vi "集成干预.vi"(11 "数据标记表":string(combo)="N") -> ()   [LabVIEW 2016, in "斯坦道多参数.lvlib"]
panel:
  out "运行状态":u16(ring) items=["空闲", "水样测试", "标样核查"]
  out "多参数运行日志":string
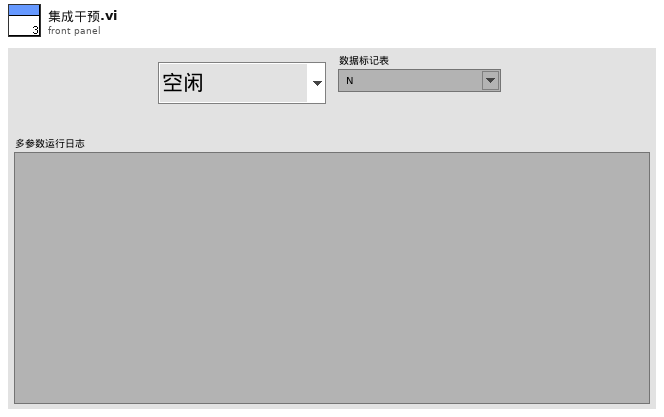
[diagram p1: front panel]
types:
  T1 = typedef "集成多参数单参数字段定义.ctl" = cluster{"时间":timestamp, "测量模式":string, "数据类型":string, "检测值":sgl, "单位":string, "数据标识":string, "标样参考值":sgl, "因子编码":string, "LastTime":timestamp}
  T2 = cluster{"水温":bool, "pH":bool, "DO":bool, "DOper":bool, "电导率":bool, "ORP":bool, "浊度":bool, "叶绿素a":bool, "藻密度":bool, "COD":bool, "DO2":bool, "DOper":bool, "氯化物":bool, "氨氮":bool, "水中油":bool}
  T3 = cluster{"ph":bool, "DO":bool, "Cond":bool, "Turb":bool, "叶绿素a":bool, "藻密度":bool, "ORP":bool, "cod":bool, "DO2":bool, "氯化物":bool, "氨氮":bool, "水中油":bool}
  T4 = cluster{"温度测量值":sgl, "测量值":sgl, "温度偏移修正值":sgl, "信号值":sgl, "数据标识":string}
  T5 = cluster{"温度测量值":sgl, "DO%":sgl, "DOmg/L":sgl, "温度偏移修正值":sgl, "数据标识mg/L":string, "数据标识%":string}
  T6 = cluster{"CH":u16, "监测值":dbl, "信号值":sgl, "数据标识":string}
  T7 = cluster{"水样数据时间":timestamp, "水温":dbl, "pH":dbl, "DO":dbl, "DOper":dbl, "电导率":dbl, "ORP":dbl, "浊度":dbl, "叶绿素a":dbl, "藻密度":dbl, "COD":dbl, "DO2":dbl, "DO2per":dbl, "氯化物":dbl, "氨氮":dbl, "水中油":dbl}
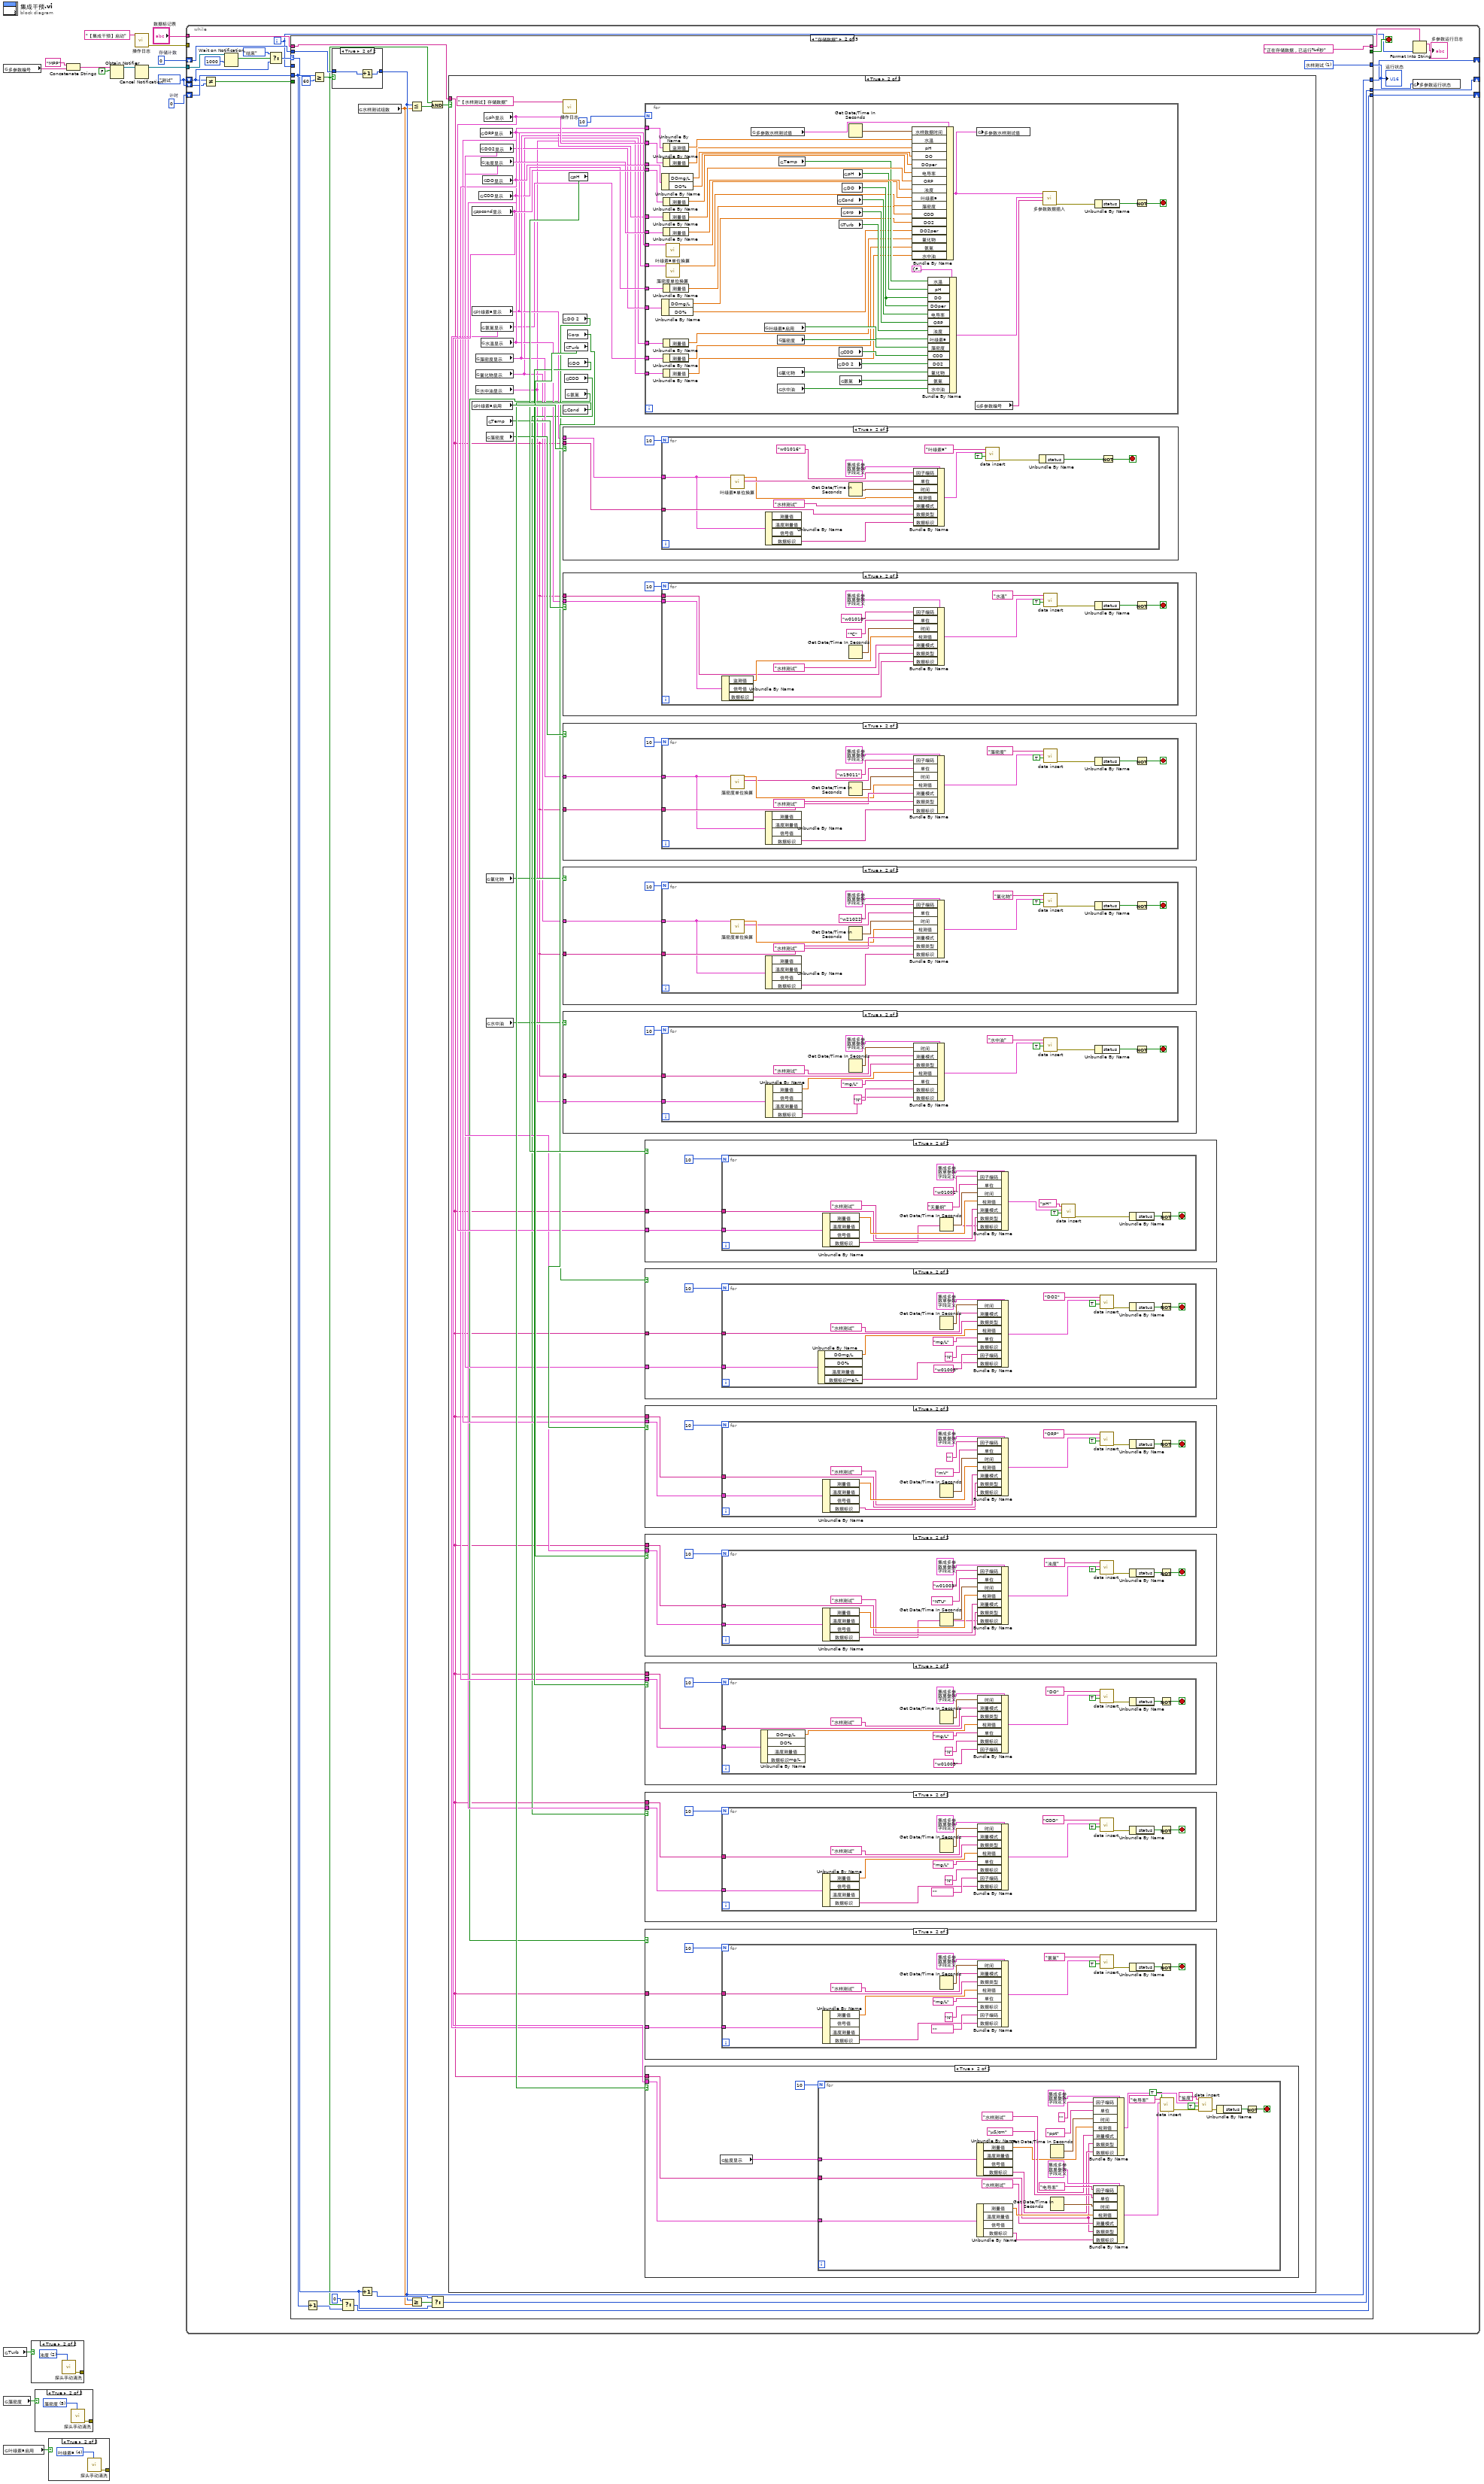
[diagram p0: block diagram]
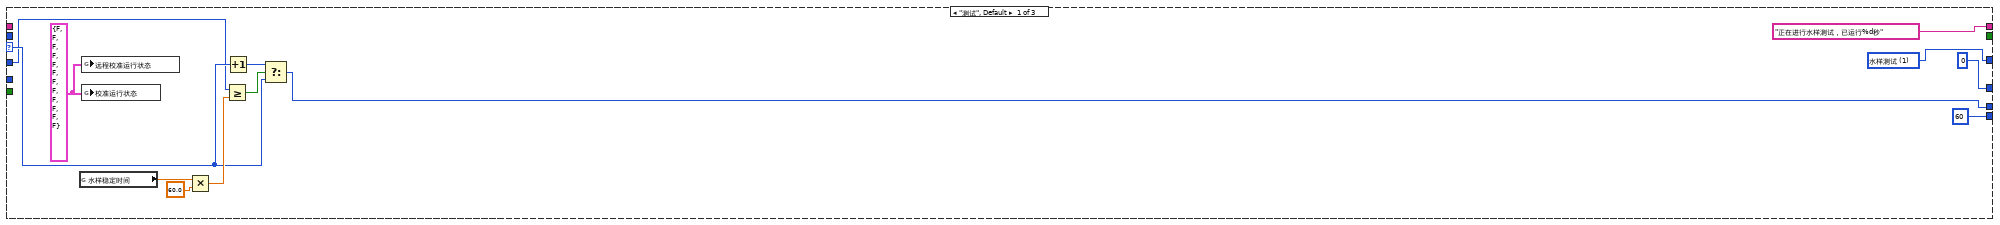
[diagram p5: hidden frame]
diagram:
  w7 = 0  # 存储计数
  w8 = 0  # 计时
  w3 = enum16{"测试", "存储数据", "结束"}."测试" ("枚举")
  n1 = global read "多参数全局变量.vi" "多参数编号"() -> (w9:string)
  n2 = global read "断电保存变量.vi" "Turb"() -> (w6:bool)
  n3 = global read "断电保存变量.vi" "藻密度"() -> (w4:bool)
  n4 = global read "断电保存变量.vi" "叶绿素a启用"() -> (w5:bool)
  n5 = case shown="True" w6 {
    tunnel: [_ w16] -> _
    frame False {
    }
    frame True {
      w17 = u16 2 items=["pH", "DO", "浊度", "电导率", "叶绿素a", "藻密度", "ORP", "DO2"] ("校准参数")
      n6 = call "探头手动清洗.vi"("校准参数"=w17) -> ("error out"=w16:errorcluster)  [unwired: 10 in]
    }
  }
  n7 = case shown="True" w4 {
    tunnel: [_ w18] -> _
    frame False {
    }
    frame True {
      w19 = u16 5 items=["pH", "DO", "浊度", "电导率", "叶绿素a", "藻密度", "ORP", "DO2"] ("校准参数")
      n8 = call "探头手动清洗.vi"("校准参数"=w19) -> ("error out"=w18:errorcluster)  [unwired: 10 in]
    }
  }
  n9 = case shown="True" w5 {
    tunnel: [_ w20] -> _
    frame False {
    }
    frame True {
      w21 = u16 4 items=["pH", "DO", "浊度", "电导率", "叶绿素a", "藻密度", "ORP", "DO2"] ("校准参数")
      n10 = call "探头手动清洗.vi"("校准参数"=w21) -> ("error out"=w20:errorcluster)  [unwired: 10 in]
    }
  }
  n11 = Concatenate Strings("MPP" ("名称（未命名）"), w9) -> (w10:string)
  n12 = Obtain Notifier(name (unnamed)=w10, notification data type=FALSE) -> (notifier out=w13:refnum<notifier>)  [unwired: 2 in, 2 out]
  n13 = call "操作日志.vi"("日志信息"="【集成干预】启动") -> ("error out"=w1:errorcluster)  [unwired: 10 in]
  n14 = Cancel Notification(0:w13) -> (8:w12:refnum<notifier>)  [unwired: 1 in, 2 out]
  n15 = while {
    shift-right: [w26] -> _
    shift-left: w3 -> [w24]
    tunnel: w12 -> [w37]
    tunnel: "数据标记表" -> [w32]
    shift-right: [w28] -> _
    shift-left: w8 -> [w30]
    shift-right: [w27] -> _
    shift-left: w7 -> [w29]
    shift-left: w3 -> [w23]
    tunnel: w1 -> [_]
    i -> [w25]
    stop <- w40 stop-if-true
    n16 = Not Equal?(x=w24, y=w23) -> (x != y?=w22:bool)
    n17 = Wait on Notification(notifier=w37, timeout in ms (-1)=1000 ("超时毫秒(-1)")) -> (notification=w35:bool)  [unwired: 2 in, 3 out]
    n18 = Select(t=enum16{"测试", "存储数据", "结束"}."结束" ("枚举"), s=w35, f=w24) -> (s? t:f=w33:enum16{"测试", "存储数据", "结束"})
    n19 = case shown="\"存储数据\"" w33 {
      selector: w33 -> [w47 w61 _]
      tunnel: [_ _ TRUE] -> w40
      tunnel: ["正在进行水样测试，已运行%d秒" ("格式字符串") "正在存储数据，已运行%d秒" ("格式字符串") "测试停止，累计运行%d秒" ("格式字符串")] -> w39
      tunnel: [w52 w66 w408] -> w31
      tunnel: w32 -> [_ w71 _]
      tunnel: w30 -> [_ w69 _]
      tunnel: w29 -> [_ w70 _]
      tunnel: [60 w54 0] -> w28
      tunnel: [0 w60 0] -> w27
      tunnel: [w45 w64 enum16{"测试", "存储数据", "结束"}."结束" ("枚举")] -> w26
      tunnel: w25 -> [w42 _ _]
      tunnel: w22 -> [_ _ w404]
      frame "测试", Default {
        w41 = T3 {"ph"=FALSE, "DO"=FALSE, "Cond"=FALSE, "Turb"=FALSE, "叶绿素a"=FALSE, "藻密度"=FALSE, "ORP"=FALSE, "cod"=FALSE, "DO2"=FALSE, "氯化物"=FALSE, "氨氮"=FALSE, "水中油"=FALSE} ("远程校准运行状态")
        w52 = u16 1 items=["空闲", "水样测试", "标样核查"] ("多参数运行状态")
        n20 = global read "断电保存变量.vi" "水样稳定时间"() -> (w51:dbl)
        n21 = global write "多参数全局变量.vi" "远程校准运行状态"(w41) -> ()
        n22 = global write "多参数全局变量.vi" "校准运行状态"(w41) -> ()
        n23 = Multiply(x=w51, y=60.0) -> (x*y=w49:dbl)
        n24 = Greater Or Equal?(x=w42, y=w49) -> (x >= y?=w48:bool)
        n25 = Increment(x=w47) -> (x+1=w46:enum16{"测试", "存储数据", "结束"})
        n26 = Select(t=w46, s=w48, f=w47) -> (s? t:f=w45:enum16{"测试", "存储数据", "结束"})
      }
      frame "存储数据" {
        w66 = u16 1 items=["空闲", "水样测试", "标样核查"] ("多参数运行状态")
        n27 = Increment(x=w69) -> (x+1=w56:i32)
        n28 = Greater Or Equal?(x=w69, y=60) -> (x >= y?=w57:bool)
        n29 = case shown="True" w57 {
          tunnel: w70 -> [w72 w74]
          tunnel: [w72 w73] -> w60
          frame False {
          }
          frame True {
            n30 = Increment(x=w74) -> (x+1=w73:i32)
          }
        }
        n31 = Select(t=0, s=w57, f=w56) -> (s? t:f=w54:i32)
        n32 = global read "断电保存变量.vi" "水样测试组数"() -> (w59:dbl)
        n33 = Increment(x=w61) -> (x+1=w62:enum16{"测试", "存储数据", "结束"})
        n34 = Less Or Equal?(x=w60, y=w59) -> (x <= y?=w65:bool)
        n35 = Greater Or Equal?(x=w60, y=w59) -> (x >= y?=w58:bool)
        n36 = And(x=w57, y=w65) -> (x .and. y?=w63:bool)
        n37 = Select(t=w62, s=w58, f=w61) -> (s? t:f=w64:enum16{"测试", "存储数据", "结束"})
        n38 = case shown="True" w63 {
          tunnel: w71 -> [_ w76]
          frame False {
          }
          frame True {
            n39 = global read "多参数全局变量.vi" "spcond显示"() -> (w94:T4)
            n40 = global read "多参数全局变量.vi" "叶绿素a显示"() -> (w88:T4)
            n41 = global read "断电保存变量.vi" "叶绿素a启用"() -> (w103:bool)
            n42 = global read "多参数全局变量.vi" "藻密度显示"() -> (w90:T4)
            n43 = global read "多参数全局变量.vi" "氯化物显示"() -> (w80:T4)
            n44 = global read "多参数全局变量.vi" "水中油显示"() -> (w75:T4)
            n45 = global read "多参数全局变量.vi" "COD显示"() -> (w85:T4)
            n46 = global read "多参数全局变量.vi" "ORP显示"() -> (w87:T4)
            n47 = global read "多参数全局变量.vi" "DO2显示"() -> (w82:T5)
            n48 = global read "多参数全局变量.vi" "浊度显示"() -> (w92:T4)
            n49 = global read "多参数全局变量.vi" "氨氮显示"() -> (w78:T4)
            n50 = global read "多参数全局变量.vi" "水温显示"() -> (w89:T6)
            n51 = global read "多参数全局变量.vi" "DO显示"() -> (w91:T5)
            n52 = global read "多参数全局变量.vi" "ph显示"() -> (w93:T4)
            n53 = global read "断电保存变量.vi" "藻密度"() -> (w97:bool)
            n54 = global read "断电保存变量.vi" "氯化物"() -> (w81:bool)
            n55 = global read "断电保存变量.vi" "水中油"() -> (w77:bool)
            n56 = global read "断电保存变量.vi" "Temp"() -> (w98:bool)
            n57 = call "操作日志.vi"("日志信息"="【水样测试】存储数据") -> ()  [unwired: 10 in, 1 out]
            n58 = global read "断电保存变量.vi" "DO 2"() -> (w83:bool)
            n59 = global read "断电保存变量.vi" "Cond"() -> (w101:bool)
            n60 = case shown="True" w103 {
              tunnel: w76 -> [_ w285]
              tunnel: w88 -> [_ w283]
              frame False {
              }
              frame True {
                n61 = for {
                  N: 10 -> [_]
                  tunnel: w285 -> [w292]
                  tunnel: w283 -> [w289]
                  stop <- w295 stop-if-true
                  n62 = call "叶绿素a单位换算.vi"("叶绿素a显示"=w289) -> ("检测值1.单位"=w288:string, "测量值"=w287:sgl)  [unwired: 8 in, 1 out]
                  n63 = Unbundle By Name(w289) -> ("数据标识"=w291:string)  [unwired: 3 out]
                  n64 = Get Date/Time In Seconds() -> (seconds since 1Jan1904=w294:timestamp)
                  n65 = Bundle By Name(cluster=T1 {"时间"=timestamp(0 s since 1904-01-01), "测量模式"="水样测试", "数据类型"="N", "检测值"=0.0, "单位"="mg/L", "数据标识"="N", "标样参考值"=0.0, "因子编码"="", "LastTime"=timestamp(0 s since 1904-01-01)} ("data"), "因子编码"="w01016", "单位"=w288, "时间"=w294, "检测值"=w287, "测量模式"="水样测试", "数据类型"=w292, "数据标识"=w291) -> (w299:T1)
                  n66 = call "data insert.vi"("集成干预"=TRUE, "data"=w299, "table in"="叶绿素a" ("table输入")) -> ("error out"=w297:errorcluster)  [unwired: 8 in]
                  n67 = Unbundle By Name(w297) -> ("status"=w296:bool)
                  n68 = Not(x=w296) -> (.not. x?=w295:bool)
                }
              }
            }
            n69 = case shown="True" w98 {
              tunnel: w76 -> [_ w388]
              tunnel: w89 -> [_ w386]
              frame False {
              }
              frame True {
                n70 = for {
                  N: 10 -> [_]
                  tunnel: w388 -> [w393]
                  tunnel: w386 -> [w392]
                  stop <- w396 stop-if-true
                  n71 = Unbundle By Name(w392) -> ("监测值"=w399:dbl, "数据标识"=w391:string)  [unwired: 1 out]
                  n72 = Get Date/Time In Seconds() -> (seconds since 1Jan1904=w395:timestamp)
                  n73 = Bundle By Name(cluster=T1 {"时间"=timestamp(0 s since 1904-01-01), "测量模式"="水样测试", "数据类型"="N", "检测值"=0.0, "单位"="mg/L", "数据标识"="N", "标样参考值"=0.0, "因子编码"="", "LastTime"=timestamp(0 s since 1904-01-01)} ("data"), "因子编码"="w01010", "单位"="℃", "时间"=w395, "检测值"=w399, "测量模式"="水样测试", "数据类型"=w393, "数据标识"=w391) -> (w402:T1)
                  n74 = call "data insert.vi"("集成干预"=TRUE, "data"=w402, "table in"="水温" ("table输入")) -> ("error out"=w398:errorcluster)  [unwired: 8 in]
                  n75 = Unbundle By Name(w398) -> ("status"=w397:bool)
                  n76 = Not(x=w397) -> (.not. x?=w396:bool)
                }
              }
            }
            n77 = case shown="True" w97 {
              tunnel: w76 -> [_ w267]
              tunnel: w90 -> [_ w265]
              frame False {
              }
              frame True {
                n78 = for {
                  N: 10 -> [_]
                  tunnel: w267 -> [w275]
                  tunnel: w265 -> [w271]
                  stop <- w276 stop-if-true
                  n79 = call "藻密度单位换算.vi"("藻密度显示"=w271) -> ("检测值1.单位"=w269:string, "测量值"=w270:sgl)  [unwired: 8 in, 1 out]
                  n80 = Unbundle By Name(w271) -> ("数据标识"=w273:string)  [unwired: 3 out]
                  n81 = Get Date/Time In Seconds() -> (seconds since 1Jan1904=w277:timestamp)
                  n82 = Bundle By Name(cluster=T1 {"时间"=timestamp(0 s since 1904-01-01), "测量模式"="水样测试", "数据类型"="N", "检测值"=0.0, "单位"="mg/L", "数据标识"="N", "标样参考值"=0.0, "因子编码"="", "LastTime"=timestamp(0 s since 1904-01-01)} ("data"), "因子编码"="w19011", "单位"=w269, "时间"=w277, "检测值"=w270, "测量模式"="水样测试", "数据类型"=w275, "数据标识"=w273) -> (w278:T1)
                  n83 = call "data insert.vi"("集成干预"=TRUE, "data"=w278, "table in"="藻密度" ("table输入")) -> ("error out"=w280:errorcluster)  [unwired: 8 in]
                  n84 = Unbundle By Name(w280) -> ("status"=w279:bool)
                  n85 = Not(x=w279) -> (.not. x?=w276:bool)
                }
              }
            }
            n86 = case shown="True" w81 {
              tunnel: w76 -> [_ w143]
              tunnel: w80 -> [_ w141]
              frame False {
              }
              frame True {
                n87 = for {
                  N: 10 -> [_]
                  tunnel: w143 -> [w153]
                  tunnel: w141 -> [w149]
                  stop <- w154 stop-if-true
                  n88 = call "藻密度单位换算.vi"("藻密度显示"=w149) -> ("检测值1.单位"=w147:string, "测量值"=w148:sgl)  [unwired: 8 in, 1 out]
                  n89 = Unbundle By Name(w149) -> ("数据标识"=w151:string)  [unwired: 3 out]
                  n90 = Get Date/Time In Seconds() -> (seconds since 1Jan1904=w155:timestamp)
                  n91 = Bundle By Name(cluster=T1 {"时间"=timestamp(0 s since 1904-01-01), "测量模式"="水样测试", "数据类型"="N", "检测值"=0.0, "单位"="mg/L", "数据标识"="N", "标样参考值"=0.0, "因子编码"="", "LastTime"=timestamp(0 s since 1904-01-01)} ("data"), "因子编码"="w21022", "单位"=w147, "时间"=w155, "检测值"=w148, "测量模式"="水样测试", "数据类型"=w153, "数据标识"=w151) -> (w156:T1)
                  n92 = call "data insert.vi"("集成干预"=TRUE, "data"=w156, "table in"="氯化物") -> ("error out"=w158:errorcluster)  [unwired: 8 in]
                  n93 = Unbundle By Name(w158) -> ("status"=w157:bool)
                  n94 = Not(x=w157) -> (.not. x?=w154:bool)
                }
              }
            }
            n95 = case shown="True" w77 {
              tunnel: w76 -> [_ w106]
              tunnel: w75 -> [_ w104]
              frame False {
              }
              frame True {
                n96 = for {
                  N: 10 -> [_]
                  tunnel: w106 -> [w118]
                  tunnel: w104 -> [w111]
                  stop <- w121 stop-if-true
                  n97 = Unbundle By Name(w111) -> ("测量值"=w110:sgl, "数据标识"=w109:string)  [unwired: 2 out]
                  n98 = Get Date/Time In Seconds() -> (seconds since 1Jan1904=w120:timestamp)
                  n99 = Bundle By Name(cluster=T1 {"时间"=timestamp(0 s since 1904-01-01), "测量模式"="水样测试", "数据类型"="N", "检测值"=0.0, "单位"="mg/L", "数据标识"="N", "标样参考值"=0.0, "因子编码"="", "LastTime"=timestamp(0 s since 1904-01-01)} ("data"), "时间"=w120, "测量模式"="水样测试", "数据类型"=w118, "检测值"=w110, "单位"="mg/L", "数据标识"="N" ("水样数据标识"), "数据标识"=w109) -> (w113:T1)
                  n100 = call "data insert.vi"("集成干预"=TRUE, "data"=w113, "table in"="水中油") -> ("error out"=w114:errorcluster)  [unwired: 8 in]
                  n101 = Unbundle By Name(w114) -> ("status"=w115:bool)
                  n102 = Not(x=w115) -> (.not. x?=w121:bool)
                }
              }
            }
            n103 = global read "断电保存变量.vi" "Turb"() -> (w102:bool)
            n104 = global read "断电保存变量.vi" "COD"() -> (w84:bool)
            n105 = global read "断电保存变量.vi" "氨氮"() -> (w79:bool)
            n106 = global read "断电保存变量.vi" "orp"() -> (w96:bool)
            n107 = global read "断电保存变量.vi" "DO"() -> (w100:bool)
            n108 = global read "断电保存变量.vi" "pH"() -> (w99:bool)
            n109 = for {
              N: 10 -> [_]
              tunnel: w89 -> [w226]
              tunnel: w93 -> [w225]
              tunnel: w91 -> [w224]
              tunnel: w94 -> [w223]
              tunnel: w87 -> [w222]
              tunnel: w92 -> [w221]
              tunnel: w88 -> [w211]
              tunnel: w90 -> [w213]
              tunnel: w85 -> [w219]
              tunnel: w82 -> [w216]
              tunnel: w80 -> [w207]
              tunnel: w78 -> [w205]
              tunnel: w75 -> [w198]
              stop <- w228 stop-if-true
              n110 = Unbundle By Name(w224) -> ("DOmg/L"=w243:sgl, "DO%"=w242:sgl)
              n111 = Unbundle By Name(w216) -> ("DOmg/L"=w215:sgl, "DO%"=w214:sgl)
              n112 = Unbundle By Name(w226) -> ("监测值"=w245:dbl)
              n113 = Unbundle By Name(w225) -> ("测量值"=w244:sgl)
              n114 = Unbundle By Name(w223) -> ("测量值"=w241:sgl)
              n115 = Unbundle By Name(w222) -> ("测量值"=w240:sgl)
              n116 = Unbundle By Name(w221) -> ("测量值"=w239:sgl)
              n117 = Unbundle By Name(w219) -> ("测量值"=w218:sgl)
              n118 = Unbundle By Name(w207) -> ("测量值"=w206:sgl)
              n119 = Unbundle By Name(w205) -> ("测量值"=w204:sgl)
              n120 = Unbundle By Name(w198) -> ("测量值"=w197:sgl)
              n121 = call "叶绿素a单位换算.vi"("叶绿素a显示"=w211) -> ("测量值"=w210:sgl)  [unwired: 8 in, 2 out]
              n122 = call "藻密度单位换算.vi"("藻密度显示"=w213) -> ("测量值"=w212:sgl)  [unwired: 8 in, 2 out]
              n123 = global read "多参数全局变量.vi" "多参数水样测试值"() -> (w202:T7)
              n124 = global read "断电保存变量.vi" "叶绿素a启用"() -> (w232:bool)
              n125 = global read "断电保存变量.vi" "藻密度"() -> (w235:bool)
              n126 = global read "断电保存变量.vi" "氯化物"() -> (w208:bool)
              n127 = global read "断电保存变量.vi" "水中油"() -> (w199:bool)
              n128 = global read "断电保存变量.vi" "Temp"() -> (w234:bool)
              n129 = global read "断电保存变量.vi" "Cond"() -> (w237:bool)
              n130 = global read "断电保存变量.vi" "DO 2"() -> (w217:bool)
              n131 = global read "断电保存变量.vi" "Turb"() -> (w236:bool)
              n132 = global read "断电保存变量.vi" "COD"() -> (w220:bool)
              n133 = global read "断电保存变量.vi" "氨氮"() -> (w203:bool)
              n134 = global read "断电保存变量.vi" "orp"() -> (w233:bool)
              n135 = global read "断电保存变量.vi" "DO"() -> (w231:bool)
              n136 = global read "断电保存变量.vi" "pH"() -> (w238:bool)
              n137 = Get Date/Time In Seconds() -> (seconds since 1Jan1904=w246:timestamp)
              n138 = Bundle By Name(cluster=w202, "水样数据时间"=w246, "水温"=w245, "pH"=w244, "DO"=w243, "DOper"=w242, "电导率"=w241, "ORP"=w240, "浊度"=w239, "叶绿素a"=w210, "藻密度"=w212, "COD"=w218, "DO2"=w215, "DO2per"=w214, "氯化物"=w206, "氨氮"=w204, "水中油"=w197) -> (w209:T7)
              n139 = Bundle By Name(cluster=T2 {"水温"=FALSE, "pH"=FALSE, "DO"=FALSE, "DOper"=FALSE, "电导率"=FALSE, "ORP"=FALSE, "浊度"=FALSE, "叶绿素a"=FALSE, "藻密度"=FALSE, "COD"=FALSE, "DO2"=FALSE, "DOper"=FALSE, "氯化物"=FALSE, "氨氮"=FALSE, "水中油"=FALSE} ("columns enable"), "水温"=w234, "pH"=w238, "DO"=w231, "DOper"=w231, "电导率"=w237, "ORP"=w233, "浊度"=w236, "叶绿素a"=w232, "藻密度"=w235, "COD"=w220, "DO2"=w217, "氯化物"=w208, "氨氮"=w203, "水中油"=w199) -> (w200:T2)
              n140 = global read "多参数全局变量.vi" "多参数编号"() -> (w227:string)
              n141 = global write "多参数全局变量.vi" "多参数水样测试值"(w209) -> ()
              n142 = call "多参数数据插入.vi"("编号"=w227, "columns enable"=w200, "data in"=w209) -> ("error out"=w230:errorcluster)  [unwired: 8 in]
              n143 = Unbundle By Name(w230) -> ("status"=w229:bool)
              n144 = Not(x=w229) -> (.not. x?=w228:bool)
            }
            n145 = case shown="True" w99 {
              tunnel: w76 -> [_ w370]
              tunnel: w93 -> [_ w368]
              frame False {
              }
              frame True {
                n146 = for {
                  N: 10 -> [_]
                  tunnel: w370 -> [w375]
                  tunnel: w368 -> [w374]
                  stop <- w378 stop-if-true
                  n147 = Unbundle By Name(w374) -> ("测量值"=w381:sgl, "数据标识"=w373:string)  [unwired: 2 out]
                  n148 = Get Date/Time In Seconds() -> (seconds since 1Jan1904=w377:timestamp)
                  n149 = Bundle By Name(cluster=T1 {"时间"=timestamp(0 s since 1904-01-01), "测量模式"="水样测试", "数据类型"="N", "检测值"=0.0, "单位"="mg/L", "数据标识"="N", "标样参考值"=0.0, "因子编码"="", "LastTime"=timestamp(0 s since 1904-01-01)} ("data"), "因子编码"="w01001", "单位"="无量纲", "时间"=w377, "检测值"=w381, "测量模式"="水样测试", "数据类型"=w375, "数据标识"=w373) -> (w385:T1)
                  n150 = call "data insert.vi"("集成干预"=TRUE, "data"=w385, "table in"="pH" ("table输入")) -> ("error out"=w380:errorcluster)  [unwired: 8 in]
                  n151 = Unbundle By Name(w380) -> ("status"=w379:bool)
                  n152 = Not(x=w379) -> (.not. x?=w378:bool)
                }
              }
            }
            n153 = case shown="True" w83 {
              tunnel: w76 -> [_ w161]
              tunnel: w82 -> [_ w159]
              frame False {
              }
              frame True {
                n154 = for {
                  N: 10 -> [_]
                  tunnel: w161 -> [w174]
                  tunnel: w159 -> [w166]
                  stop <- w177 stop-if-true
                  n155 = Unbundle By Name(w166) -> ("DOmg/L"=w173:sgl, "数据标识mg/L"=w165:string)  [unwired: 2 out]
                  n156 = Get Date/Time In Seconds() -> (seconds since 1Jan1904=w176:timestamp)
                  n157 = Bundle By Name(cluster=T1 {"时间"=timestamp(0 s since 1904-01-01), "测量模式"="水样测试", "数据类型"="N", "检测值"=0.0, "单位"="mg/L", "数据标识"="N", "标样参考值"=0.0, "因子编码"="", "LastTime"=timestamp(0 s since 1904-01-01)} ("data"), "时间"=w176, "测量模式"="水样测试", "数据类型"=w174, "检测值"=w173, "单位"="mg/L", "数据标识"="N" ("水样数据标识"), "因子编码"="w01009", "数据标识"=w165) -> (w167:T1)
                  n158 = call "data insert.vi"("集成干预"=TRUE, "data"=w167, "table in"="DO2") -> ("error out"=w169:errorcluster)  [unwired: 8 in]
                  n159 = Unbundle By Name(w169) -> ("status"=w170:bool)
                  n160 = Not(x=w170) -> (.not. x?=w177:bool)
                }
              }
            }
            n161 = case shown="True" w96 {
              tunnel: w76 -> [_ w249]
              tunnel: w87 -> [_ w247]
              frame False {
              }
              frame True {
                n162 = for {
                  N: 10 -> [_]
                  tunnel: w249 -> [w256]
                  tunnel: w247 -> [w254]
                  stop <- w258 stop-if-true
                  n163 = Unbundle By Name(w254) -> ("测量值"=w264:sgl, "数据标识"=w253:string)  [unwired: 2 out]
                  n164 = Get Date/Time In Seconds() -> (seconds since 1Jan1904=w257:timestamp)
                  n165 = Bundle By Name(cluster=T1 {"时间"=timestamp(0 s since 1904-01-01), "测量模式"="水样测试", "数据类型"="N", "检测值"=0.0, "单位"="mg/L", "数据标识"="N", "标样参考值"=0.0, "因子编码"="", "LastTime"=timestamp(0 s since 1904-01-01)} ("data"), "因子编码"="", "单位"="mV", "时间"=w257, "检测值"=w264, "测量模式"="水样测试", "数据类型"=w256, "数据标识"=w253) -> (w251:T1)
                  n166 = call "data insert.vi"("集成干预"=TRUE, "data"=w251, "table in"="ORP" ("table输入")) -> ("error out"=w261:errorcluster)  [unwired: 8 in]
                  n167 = Unbundle By Name(w261) -> ("status"=w260:bool)
                  n168 = Not(x=w260) -> (.not. x?=w258:bool)
                }
              }
            }
            n169 = case shown="True" w102 {
              tunnel: w76 -> [_ w303]
              tunnel: w92 -> [_ w301]
              frame False {
              }
              frame True {
                n170 = for {
                  N: 10 -> [_]
                  tunnel: w303 -> [w308]
                  tunnel: w301 -> [w307]
                  stop <- w311 stop-if-true
                  n171 = Unbundle By Name(w307) -> ("测量值"=w314:sgl, "数据标识"=w306:string)  [unwired: 2 out]
                  n172 = Get Date/Time In Seconds() -> (seconds since 1Jan1904=w310:timestamp)
                  n173 = Bundle By Name(cluster=T1 {"时间"=timestamp(0 s since 1904-01-01), "测量模式"="水样测试", "数据类型"="N", "检测值"=0.0, "单位"="mg/L", "数据标识"="N", "标样参考值"=0.0, "因子编码"="", "LastTime"=timestamp(0 s since 1904-01-01)} ("data"), "因子编码"="w01003", "单位"="NTU", "时间"=w310, "检测值"=w314, "测量模式"="水样测试", "数据类型"=w308, "数据标识"=w306) -> (w317:T1)
                  n174 = call "data insert.vi"("集成干预"=TRUE, "data"=w317, "table in"="浊度" ("table输入")) -> ("error out"=w313:errorcluster)  [unwired: 8 in]
                  n175 = Unbundle By Name(w313) -> ("status"=w312:bool)
                  n176 = Not(x=w312) -> (.not. x?=w311:bool)
                }
              }
            }
            n177 = case shown="True" w100 {
              tunnel: w76 -> [_ w352]
              tunnel: w91 -> [_ w350]
              frame False {
              }
              frame True {
                n178 = for {
                  N: 10 -> [_]
                  tunnel: w352 -> [w363]
                  tunnel: w350 -> [w356]
                  stop <- w367 stop-if-true
                  n179 = Unbundle By Name(w356) -> ("DOmg/L"=w362:sgl)  [unwired: 3 out]
                  n180 = Get Date/Time In Seconds() -> (seconds since 1Jan1904=w365:timestamp)
                  n181 = Bundle By Name(cluster=T1 {"时间"=timestamp(0 s since 1904-01-01), "测量模式"="水样测试", "数据类型"="N", "检测值"=0.0, "单位"="mg/L", "数据标识"="N", "标样参考值"=0.0, "因子编码"="", "LastTime"=timestamp(0 s since 1904-01-01)} ("data"), "时间"=w365, "测量模式"="水样测试", "数据类型"=w363, "检测值"=w362, "单位"="mg/L", "数据标识"="N", "因子编码"="w01009") -> (w357:T1)
                  n182 = call "data insert.vi"("集成干预"=TRUE, "data"=w357, "table in"="DO") -> ("error out"=w359:errorcluster)  [unwired: 8 in]
                  n183 = Unbundle By Name(w359) -> ("status"=w360:bool)
                  n184 = Not(x=w360) -> (.not. x?=w367:bool)
                }
              }
            }
            n185 = case shown="True" w84 {
              tunnel: w76 -> [_ w180]
              tunnel: w85 -> [_ w178]
              frame False {
              }
              frame True {
                n186 = for {
                  N: 10 -> [_]
                  tunnel: w180 -> [w192]
                  tunnel: w178 -> [w184]
                  stop <- w196 stop-if-true
                  n187 = Unbundle By Name(w184) -> ("测量值"=w191:sgl, "数据标识"=w183:string)  [unwired: 2 out]
                  n188 = Get Date/Time In Seconds() -> (seconds since 1Jan1904=w194:timestamp)
                  n189 = Bundle By Name(cluster=T1 {"时间"=timestamp(0 s since 1904-01-01), "测量模式"="水样测试", "数据类型"="N", "检测值"=0.0, "单位"="mg/L", "数据标识"="N", "标样参考值"=0.0, "因子编码"="", "LastTime"=timestamp(0 s since 1904-01-01)} ("data"), "时间"=w194, "测量模式"="水样测试", "数据类型"=w192, "检测值"=w191, "单位"="mg/L", "数据标识"="N" ("水样数据标识"), "因子编码"="", "数据标识"=w183) -> (w185:T1)
                  n190 = call "data insert.vi"("集成干预"=TRUE, "data"=w185, "table in"="COD") -> ("error out"=w187:errorcluster)  [unwired: 8 in]
                  n191 = Unbundle By Name(w187) -> ("status"=w188:bool)
                  n192 = Not(x=w188) -> (.not. x?=w196:bool)
                }
              }
            }
            n193 = case shown="True" w79 {
              tunnel: w76 -> [_ w124]
              tunnel: w78 -> [_ w122]
              frame False {
              }
              frame True {
                n194 = for {
                  N: 10 -> [_]
                  tunnel: w124 -> [w136]
                  tunnel: w122 -> [w128]
                  stop <- w140 stop-if-true
                  n195 = Unbundle By Name(w128) -> ("测量值"=w127:sgl, "数据标识"=w126:string)  [unwired: 2 out]
                  n196 = Get Date/Time In Seconds() -> (seconds since 1Jan1904=w138:timestamp)
                  n197 = Bundle By Name(cluster=T1 {"时间"=timestamp(0 s since 1904-01-01), "测量模式"="水样测试", "数据类型"="N", "检测值"=0.0, "单位"="mg/L", "数据标识"="N", "标样参考值"=0.0, "因子编码"="", "LastTime"=timestamp(0 s since 1904-01-01)} ("data"), "时间"=w138, "测量模式"="水样测试", "数据类型"=w136, "检测值"=w127, "单位"="mg/L", "数据标识"="N" ("水样数据标识"), "因子编码"="", "数据标识"=w126) -> (w130:T1)
                  n198 = call "data insert.vi"("集成干预"=TRUE, "data"=w130, "table in"="氨氮") -> ("error out"=w132:errorcluster)  [unwired: 8 in]
                  n199 = Unbundle By Name(w132) -> ("status"=w133:bool)
                  n200 = Not(x=w133) -> (.not. x?=w140:bool)
                }
              }
            }
            n201 = case shown="True" w101 {
              tunnel: w76 -> [_ w322]
              tunnel: w94 -> [_ w320]
              frame False {
              }
              frame True {
                n202 = global read "多参数全局变量.vi" "盐度显示"() -> (w319:T4)
                n203 = for {
                  N: 10 -> [_]
                  tunnel: w322 -> [w330]
                  tunnel: w320 -> [w340]
                  tunnel: w319 -> [w329]
                  stop <- w344 stop-if-true
                  n204 = Unbundle By Name(w329) -> ("测量值"=w331:sgl, "数据标识"=w336:string)  [unwired: 2 out]
                  n205 = Unbundle By Name(w340) -> ("测量值"=w347:sgl, "数据标识"=w339:string)  [unwired: 2 out]
                  n206 = Get Date/Time In Seconds() -> (seconds since 1Jan1904=w333:timestamp)
                  n207 = Get Date/Time In Seconds() -> (seconds since 1Jan1904=w343:timestamp)
                  n208 = Bundle By Name(cluster=T1 {"时间"=timestamp(0 s since 1904-01-01), "测量模式"="水样测试", "数据类型"="N", "检测值"=0.0, "单位"="mg/L", "数据标识"="N", "标样参考值"=0.0, "因子编码"="", "LastTime"=timestamp(0 s since 1904-01-01)} ("data"), "因子编码"="", "单位"="ppt", "时间"=w333, "检测值"=w331, "测量模式"="水样测试", "数据类型"=w330, "数据标识"=w336) -> (w335:T1)
                  n209 = Bundle By Name(cluster=T1 {"时间"=timestamp(0 s since 1904-01-01), "测量模式"="水样测试", "数据类型"="N", "检测值"=0.0, "单位"="mg/L", "数据标识"="N", "标样参考值"=0.0, "因子编码"="", "LastTime"=timestamp(0 s since 1904-01-01)} ("data"), "因子编码"="电导率", "单位"="μS/cm", "时间"=w343, "检测值"=w347, "测量模式"="水样测试", "数据类型"=w330, "数据标识"=w339) -> (w341:T1)
                  n210 = call "data insert.vi"("集成干预"=TRUE, "data"=w341, "table in"="电导率" ("table输入")) -> ("error out"=w326:errorcluster)  [unwired: 8 in]
                  n211 = call "data insert.vi"("error in (no error)"=w326, "集成干预"=TRUE, "data"=w335, "table in"="盐度") -> ("error out"=w325:errorcluster)  [unwired: 7 in]
                  n212 = Unbundle By Name(w325) -> ("status"=w346:bool)
                  n213 = Not(x=w346) -> (.not. x?=w344:bool)
                }
              }
            }
          }
        }
      }
      frame "结束" {
        w408 = u16 0 items=["空闲", "水样测试", "标样核查"] ("多参数运行状态")
        n214 = case shown="True" w404 {
          frame False {
          }
          frame True {
            n215 = call "操作日志.vi"("日志信息"="【集成干预】结束") -> ()  [unwired: 10 in, 1 out]
          }
        }
      }
    }
    "运行状态" <- w31
    n216 = Format Into String(format string=w39, w25) -> (resulting string=→"多参数运行日志":string)  [unwired: 2 in, 1 out]
    n217 = global write "多参数全局变量.vi" "多参数运行状态"(w31) -> ()
  }
